vi "EditOptions.vi"(8 "error in":errorcluster, 11 "node in":refnum<class "CustomDevice.lvclass">) -> (0 "error out":errorcluster, 1 "edit options":T1, 2 "subnodes class":T2, 3 "node out":refnum<class "CustomDevice.lvclass">)   [LabVIEW 2015, in "CustomDevice.lvclass"]
doc: "Contains the options for the Menu that will be displayed when doing right click on an item.\nThe sub nodes class configures which nodes can be added to this nodes\nAnd the edit options determine which options are available for the node.\nThis configuration is stored in this VI in case some dynamic configuration is required for the menu options or sub nodes."
uses:
  CustomDevice.lvclass
  <vilib>/NI/Configuration Framework/Node/SubNodeCluster.ctl
  <vilib>/NI/Configuration Framework/Node/NodeMenuOptions.ctl
  <vilib>/NI/Configuration Framework/Node/NISE_CEF_Node.lvclass
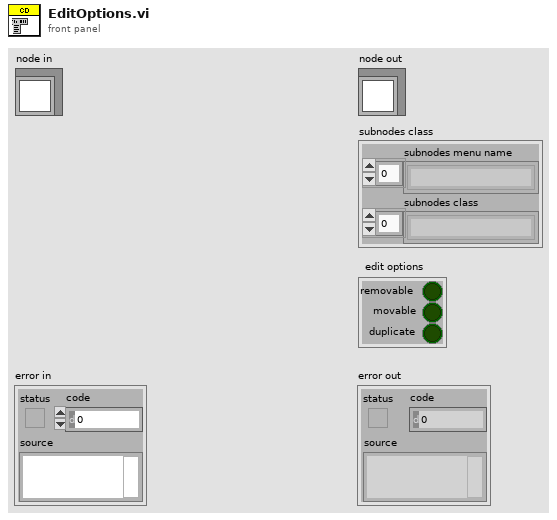
[diagram p1: front panel]
types:
  T1 = typedef "NISE_CEF_Node.lvclass/NodeMenuOptions.ctl" = cluster{"removable":bool, "movable":bool, "duplicate":bool}
  T2 = typedef "NISE_CEF_Node.lvclass/SubNodeCluster.ctl" = cluster{"subnodes menu name":string[], "subnodes class":string[]}
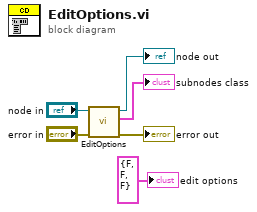
[diagram p0: block diagram]
diagram:
  n1 = call-parent "EditOptions.vi"("error in"="error in", "node in"="node in") -> ("error out"=→"error out":errorcluster, "subnodes class"=→"subnodes class":T2, "node out"=→"node out":refnum<class "CustomDevice.lvclass">)  [unwired: 6 in, 1 out]
  "edit options" <- T1 {"removable"=FALSE, "movable"=FALSE, "duplicate"=FALSE} ("edit options")
